vi "IfSyncedCompatible.vi"(8 "error in (no error)":errorcluster, 9 "Sample Rate":dbl, 10 "Frame Rate":dbl, 11 "Enum":enum16{"NoSync", "Sync"}(ring)) -> (0 "error out":errorcluster)   [LabVIEW 2023]
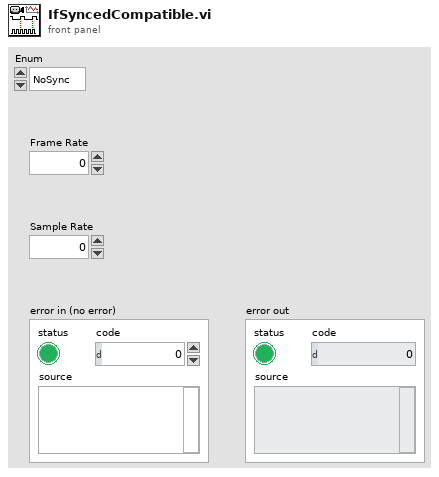
[diagram p1: front panel]
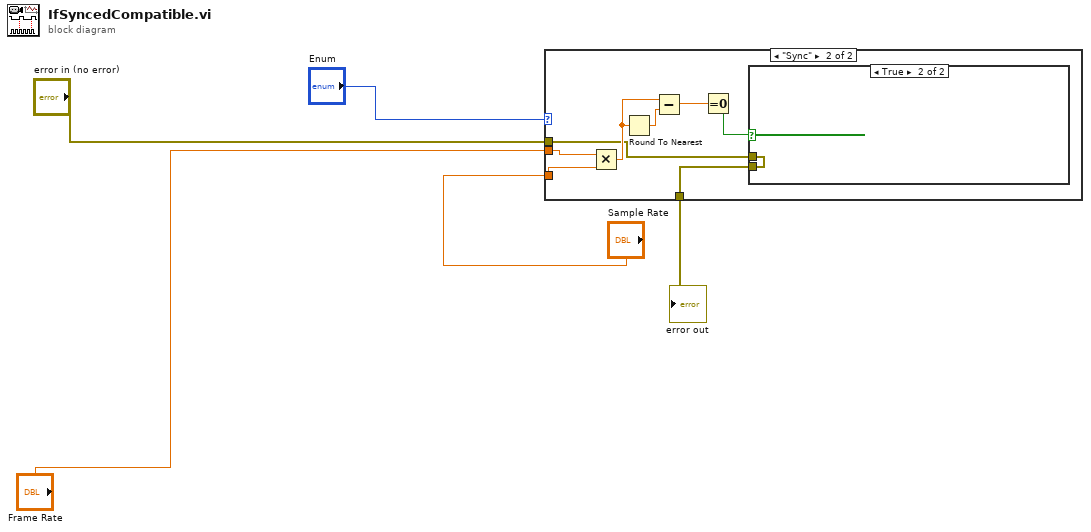
[diagram p0: block diagram]
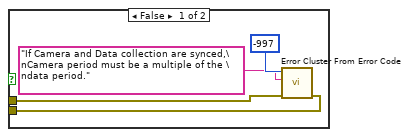
[diagram p3: hidden frame]
diagram:
  n1 = case shown="\"Sync\"" "Enum" {
    tunnel: "Frame Rate" -> [_ w14]
    tunnel: "Sample Rate" -> [_ w13]
    tunnel: "error in (no error)" -> [w6 w8]
    tunnel: [w6 w7] -> w5
    frame "NoSync", Default {
    }
    frame "Sync" {
      n2 = Multiply(x=w14, y=w13) -> (x*y=w10:dbl)
      n3 = Round To Nearest(number=w10) -> (nearest integer value=w12:dbl)
      n4 = Subtract(x=w10, y=w12) -> (x-y=w11:dbl)
      n5 = Equal To 0?(x=w11) -> (x = 0?=w9:bool)
      n6 = case shown="True" w9 {
        tunnel: w8 -> [w16 w19]
        tunnel: [w15 w19] -> w7
        frame False {
          n7 = call <vilib>:"Error Cluster From Error Code.vi"("error in (no error)"=w16, "error message (\"\")"="If Camera and Data collection are synced,\nCamera period must be a multiple of the \ndata period." ("error message (\"\")"), "error code (0)"=-997) -> ("error out"=w15:errorcluster)  [unwired: 6 in]
        }
        frame True {
        }
      }
    }
  }
  "error out" <- w5
